vi "Task 1.vi"() -> ()   [LabVIEW 2017]
panel:
  in  "stop":bool
  out "Sine 2":dynamicdata(graph) caption="Sine"
  out "Sine":dynamicdata(graph)
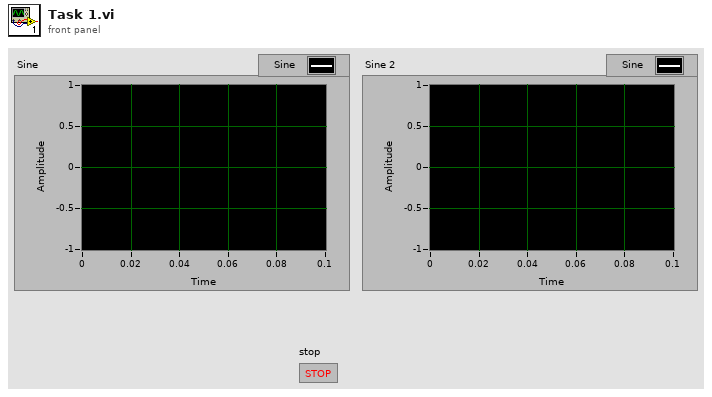
[diagram p1: front panel]
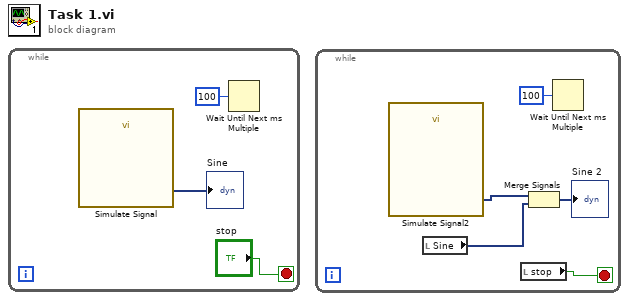
[diagram p0: block diagram]
diagram:
  n1 = while {
    stop <- "stop" stop-if-true
    n2 = call "Simulate Signal"() -> ("Sine"=→"Sine":dynamicdata)  [unwired: 14 in, 1 out]
    n3 = Wait Until Next ms Multiple(millisecond multiple=u32 100) -> ()  [unwired: 1 out]
  }
  n4 = while {
    stop <- w7 stop-if-true
    n5 = call "Simulate Signal2"() -> ("Sine"=w6:dynamicdata)  [unwired: 14 in, 1 out]
    n6 = local read "Sine"() -> (w4:dynamicdata)
    n7 = local read "stop"() -> (w7:bool)
    n8 = Merge Signals(w6, w4) -> (→"Sine 2":dynamicdata)
    n9 = Wait Until Next ms Multiple(millisecond multiple=u32 100) -> ()  [unwired: 1 out]
  }
